vi "Python.vi"() -> ()   [LabVIEW 2014]
uses:
  Controls/Standard Action.ctl
  Controls/StageStates.ctl
  <vilib>/Analysis/baseanly.llb/Mean (DBL).vi
  <vilib>/Analysis/NI_AALBase.lvlib
panel:
  out "queue":string
  out "standard output":string
  out "standard error":string
  in  "port":i32=8900
  in  "hostname":string="localhost"
  out "DM1":dbl[][](graph)
  out "DM0":dbl[][](graph)
  out "Image 2":sgl[][](graph)
  in  "launch_python":bool=TRUE
  in  "script name":string="sensorless.py"
  in  "arguments":string="nelder-mead"
  in  "Run Python":bool
  in  "Exit":bool
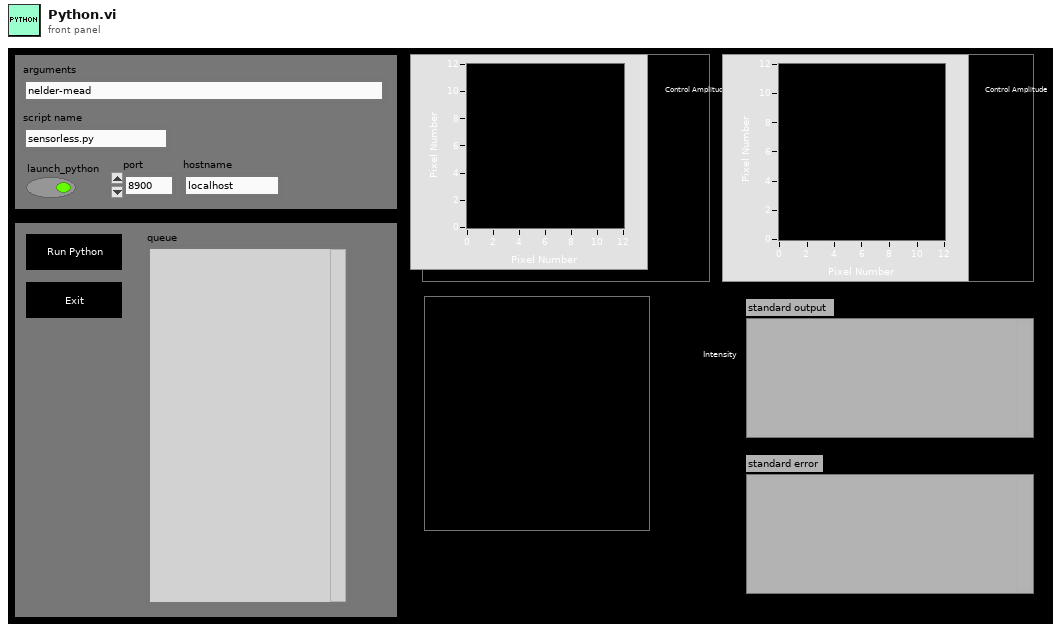
[diagram p1: front panel]
types:
  T1 = typedef "Standard Action.ctl" = enum16{"Read", "Write"}
  T2 = typedef "StageStates.ctl" = enum16{"POSITION", "MVR", "MOVE", "HALT", "ONTARGET", "ERROR", "EXIT", "HOME", "ZEROPOS", "NANOPOS", "QUIT", "ANALOG"}
  T3 = typedef "MirrorModes_DUAL.ctl" = cluster{"Mode":string, "Amplitude":dbl}[][]
  T4 = typedef "Image Acquisition Parameters.ctl" = cluster{"Scan Type":enum16{"Sample Scanning", "Beam Scanning"}, "Scan Mode":enum16{"XY", "XZ", "YZ", "XYZ"}, "Fast Axis Frequency (Hz)":dbl, "Image Format":u16, "Line Accumulations":u16, "Frames Per Capture":u16, "Frames Accumulations":u16, "Image Dimension (um)":dbl[], "Number of Z Steps":u8, "Z Steps Size (um)":dbl, "Pixel Size (nm)":dbl[], "Customized Image Format":dbl[]}
  T5 = typedef "Detectors.ctl" = cluster{"PMT":bool, "Far Red (685/40 nm)":bool, "Orange (624/40 nm)":bool, "Green (525/50 nm)":bool, "Sum All":bool}
  T6 = typedef "Laser Controls.ctl" = cluster{"STED Power (V)":dbl, "STED":bool, "650 nm":bool, "590 nm":bool, "485 nm":bool, "Manual Control":bool}
  T7 = cluster{"dm0":dbl[], "dm1":dbl[], "zcomp":dbl, "stack":sgl[][]}
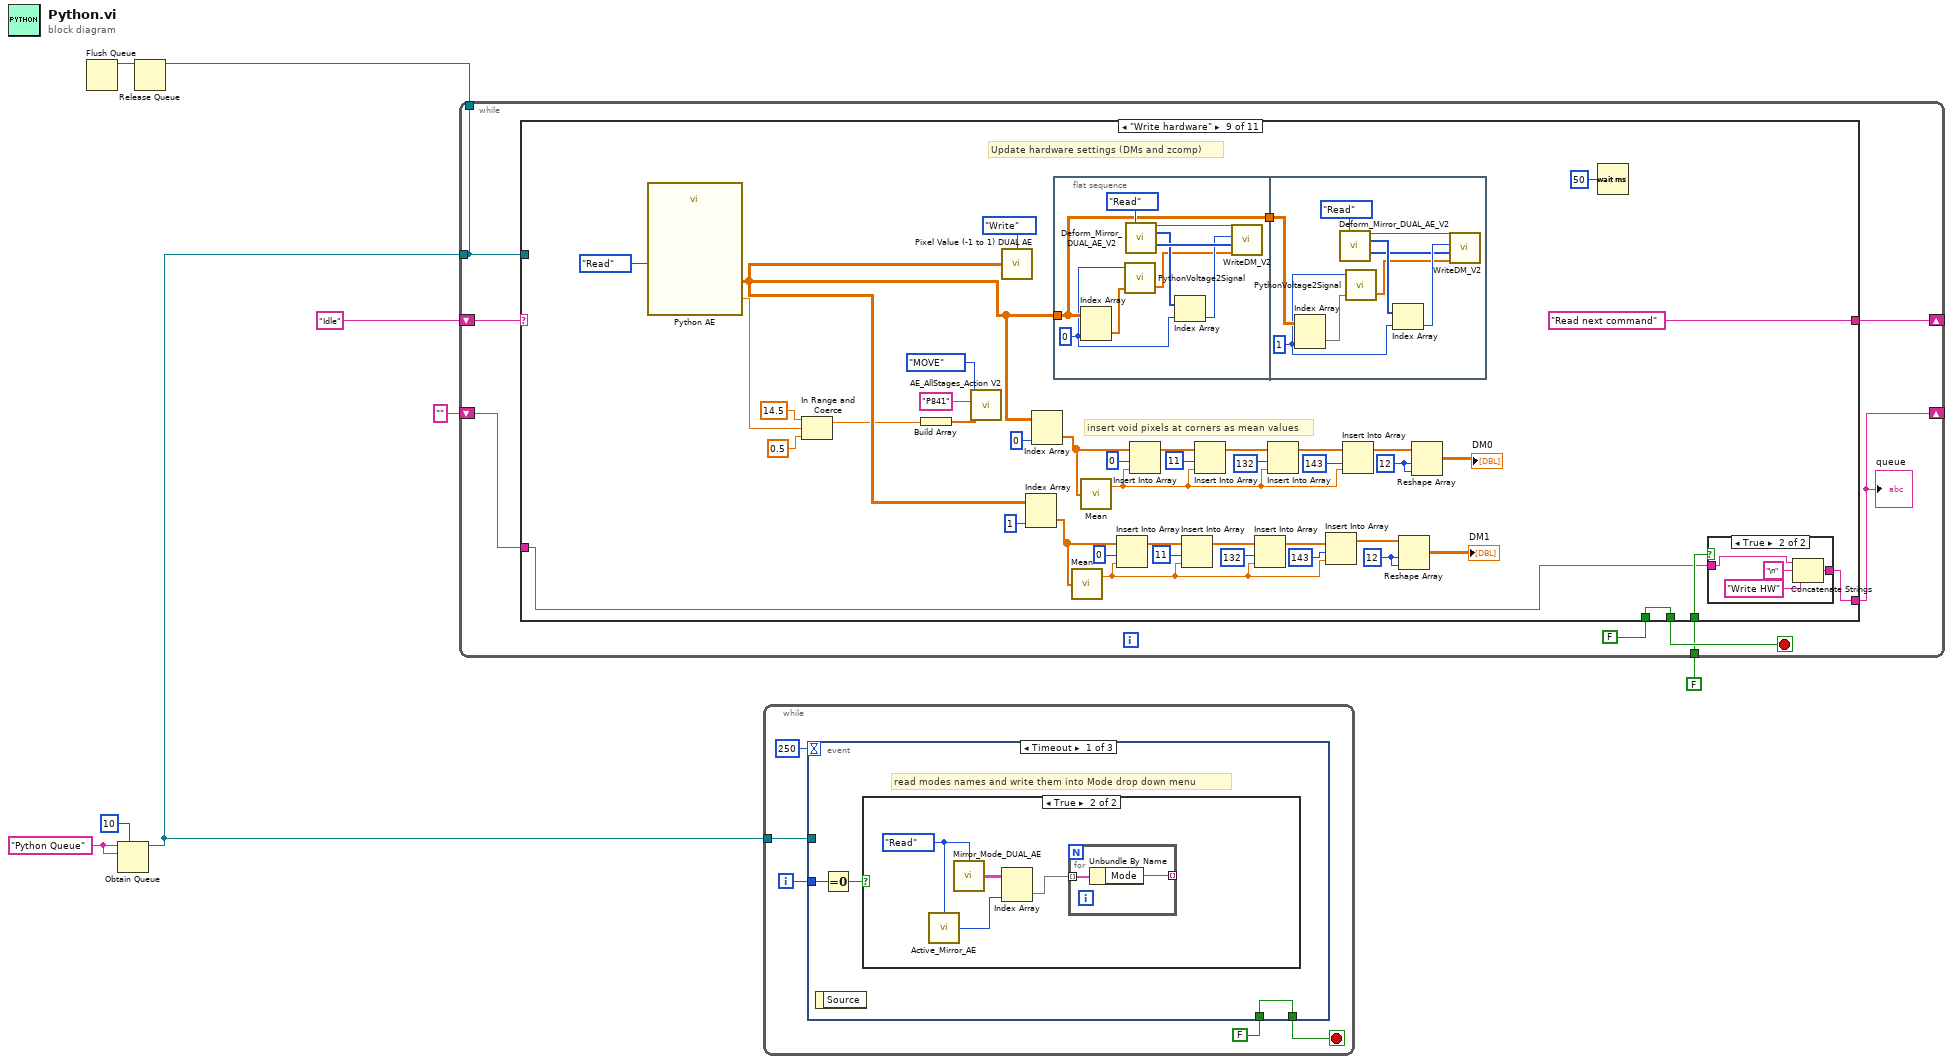
[diagram p0: block diagram]
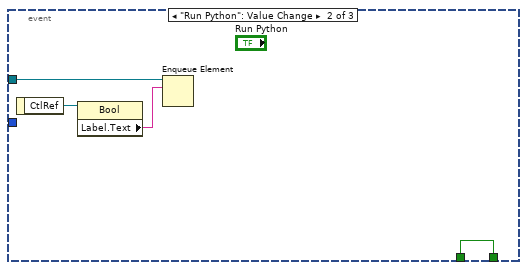
[diagram p3: hidden frame]
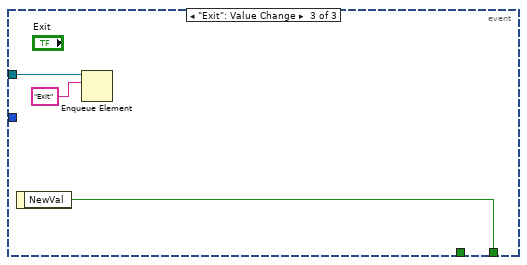
[diagram p4: hidden frame]
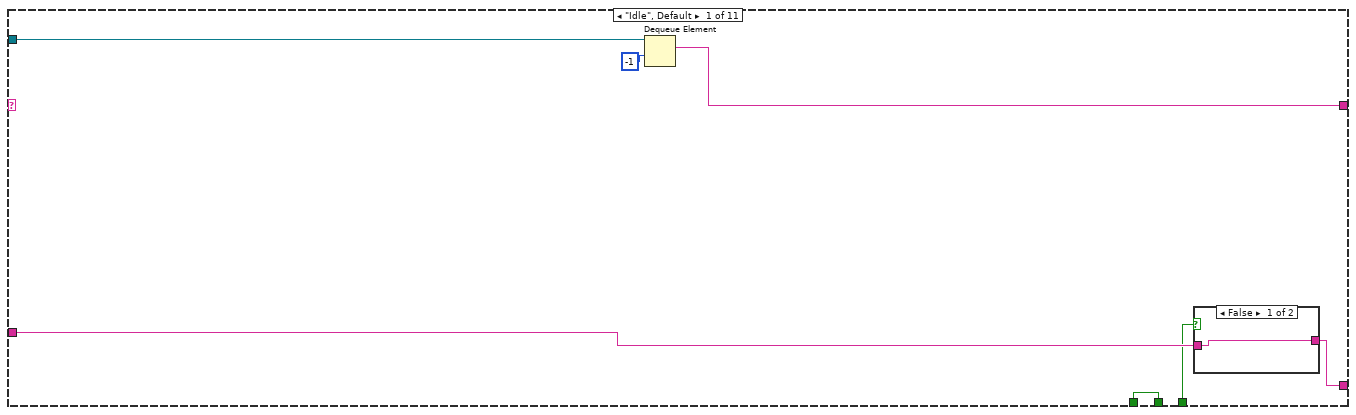
[diagram p5: hidden frame]
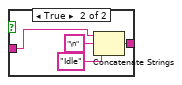
[diagram p6: hidden frame]
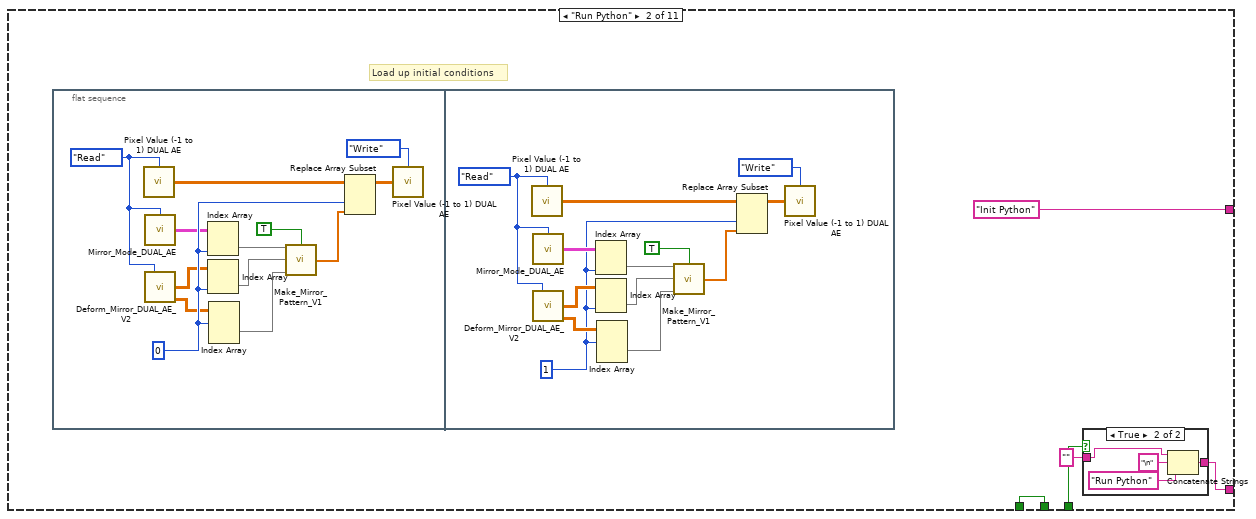
[diagram p7: hidden frame]
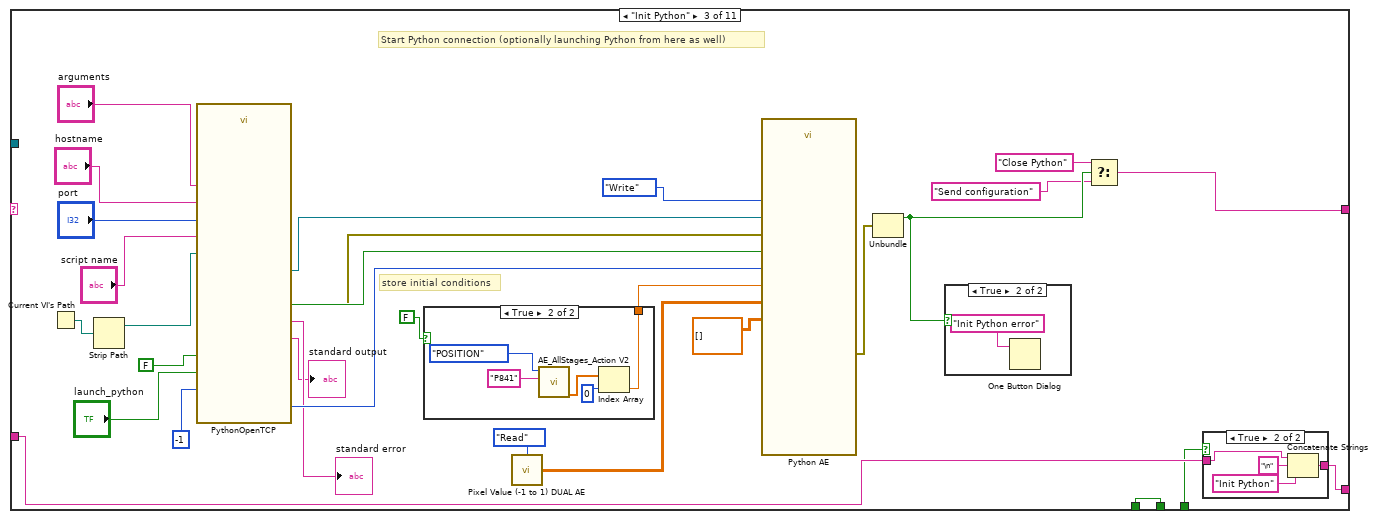
[diagram p9: hidden frame]
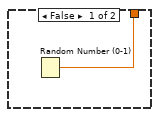
[diagram p11: hidden frame]
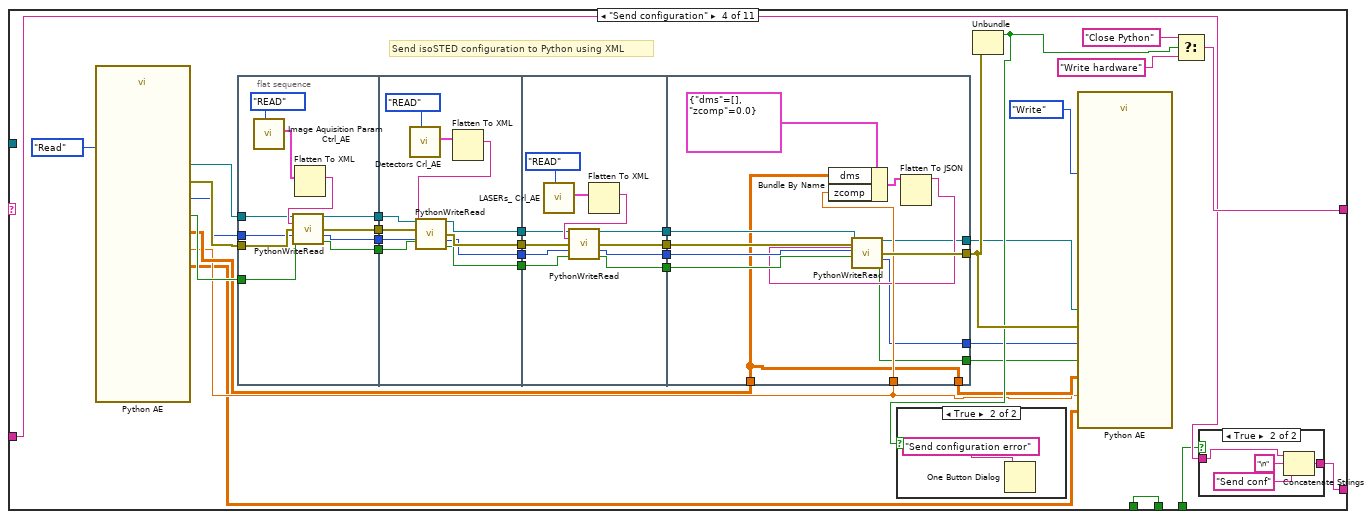
[diagram p13: hidden frame]
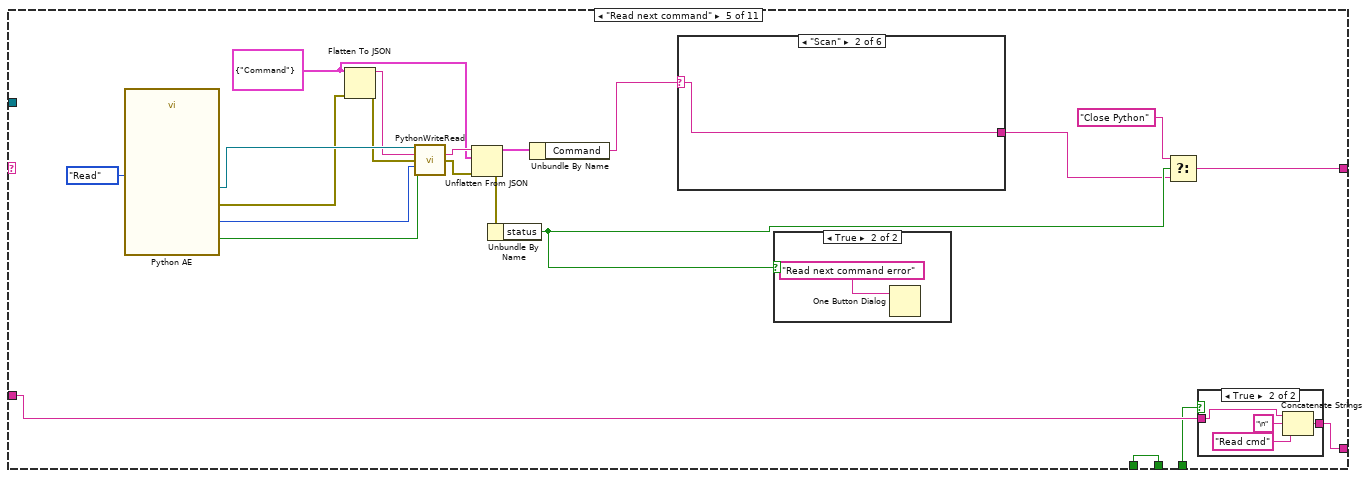
[diagram p16: hidden frame]
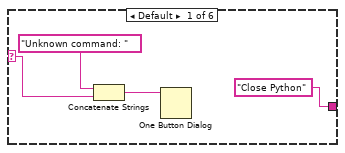
[diagram p18: hidden frame]
diagram:
  w7 = "Python Queue" ("name (unnamed)")
  n1 = Obtain Queue(max queue size (-1, unlimited)=10, name (unnamed)=w7, element data type=w7) -> (queue out=w5:refnum<queue>)  [unwired: 2 in, 2 out]
  n2 = while {
    shift-right: [w11] -> _
    shift-left: "Idle" -> [w13]
    tunnel: w5 -> [w15]
    tunnel: [w15] -> w4
    shift-right: [w10] -> _
    shift-left: "" -> [w12]
    tunnel: FALSE -> [w9]
    stop <- w16 stop-if-true
    n3 = case shown="\"Write hardware\"" w13 {
      tunnel: [w20 w33 w82 w121 w212 w249 w272 w333 w366 w435 TRUE] -> w16
      tunnel: w15 -> [w22 _ _ _ _ _ _ _ _ _ _]
      tunnel: [w21 "Init Python" ("name (unnamed)") w70 w118 w197 w233 "Python pipe" ("name (unnamed)") w334 "Read next command" ("name (unnamed)") "Idle" ("name (unnamed)") "Exit" ("name (unnamed)")] -> w11
      tunnel: FALSE -> [w20 w33 w82 w121 w212 w249 w272 w333 w366 w435 _]
      tunnel: w12 -> [w19 _ w67 w109 w195 w230 w256 w320 w359 w422 w443]
      tunnel: [w17 w31 w66 w108 w194 w231 w258 w321 w358 w421 w444] -> w10
      tunnel: w9 -> [w18 w30 w65 w107 w193 w229 w257 w319 w360 w420 w442]
      frame "Idle", Default {
        n4 = Dequeue Element(queue=w22, timeout in ms (-1)=-1) -> (element=w21:string)  [unwired: 1 in, 3 out]
        n5 = case shown="False" w18 {
          tunnel: [w24 w26] -> w17
          tunnel: w19 -> [w24 w25]
          frame False {
          }
          frame True {
            n6 = Concatenate Strings(w25, "\n" ("string"), "Idle" ("string")) -> (w26:string)
          }
        }
      }
      frame "Run Python" {
        # "Load up initial conditions"
        n7 = flat-sequence {
          frame #0 {
            w51 = 0 ("index (col)")
            w47 = Standard_Action."Read" ("Action")
            n8 = call "Pixel Value (-1 to 1) DUAL AE.vi"("Action"=w47) -> ("Pixel Value (-1 to 1) Out"=w48:dbl[][])  [unwired: 14 in]
            n9 = call "Mirror_Mode_DUAL_AE.vi"("Action"=w47) -> ("Mirror Modes Out"=w44:T3)  [unwired: 14 in]
            n10 = call "Deform_Mirror_DUAL_AE_V2.vi"("Action"=w47) -> ("Flat Files Out"=w42:dbl[][], "Mode Matrix Out"=w40:dbl[][][])  [unwired: 10 in, 3 out]
            n11 = Index Array(array=w44, index (col)=w51) -> (element=w45:cluster{"Mode":string, "Amplitude":dbl}[])  [unwired: 1 in]
            n12 = Index Array(array=w42, index (col)=w51) -> (element=w43:dbl[])  [unwired: 1 in]
            n13 = Index Array(array=w40, index (dim 0)=w51) -> (element=w39:dbl[][])  [unwired: 2 in]
            n14 = call "Make_Mirror_Pattern_V1.vi"("Mirror Modes In"=w45, "Flat On?"=TRUE ("Apply Flat"), "Flat File In"=w43, "Mirror Modes Array"=w39) -> ("Pixel Value U (-1 to 1)"=w49:dbl[])  [unwired: 11 in]
            n15 = Replace Array Subset(array=w48, new element=w49, index (col)=w51) -> (w50:dbl[][])  [unwired: 1 in]
            n16 = call "Pixel Value (-1 to 1) DUAL AE.vi"("Action"=Standard_Action."Write", "Pixel Value (-1 to 1)"=w50) -> ()  [unwired: 13 in, 1 out]
          }
          frame #1 {
            w52 = 1 ("index (col)")
            w56 = Standard_Action."Read" ("Action")
            n17 = call "Pixel Value (-1 to 1) DUAL AE.vi"("Action"=w56) -> ("Pixel Value (-1 to 1) Out"=w55:dbl[][])  [unwired: 14 in]
            n18 = call "Mirror_Mode_DUAL_AE.vi"("Action"=w56) -> ("Mirror Modes Out"=w59:T3)  [unwired: 14 in]
            n19 = call "Deform_Mirror_DUAL_AE_V2.vi"("Action"=w56) -> ("Flat Files Out"=w61:dbl[][], "Mode Matrix Out"=w63:dbl[][][])  [unwired: 10 in, 3 out]
            n20 = Index Array(array=w59, index (col)=w52) -> (element=w58:cluster{"Mode":string, "Amplitude":dbl}[])  [unwired: 1 in]
            n21 = Index Array(array=w61, index (col)=w52) -> (element=w60:dbl[])  [unwired: 1 in]
            n22 = Index Array(array=w63, index (dim 0)=w52) -> (element=w64:dbl[][])  [unwired: 2 in]
            n23 = call "Make_Mirror_Pattern_V1.vi"("Mirror Modes In"=w58, "Flat On?"=TRUE ("Apply Flat"), "Flat File In"=w60, "Mirror Modes Array"=w64) -> ("Pixel Value U (-1 to 1)"=w54:dbl[])  [unwired: 11 in]
            n24 = Replace Array Subset(array=w55, new element=w54, index (col)=w52) -> (w53:dbl[][])  [unwired: 1 in]
            n25 = call "Pixel Value (-1 to 1) DUAL AE.vi"("Action"=Standard_Action."Write", "Pixel Value (-1 to 1)"=w53) -> ()  [unwired: 13 in, 1 out]
          }
        }
        n26 = case shown="True" w30 {
          tunnel: [w34 w36] -> w31
          tunnel: "" -> [w34 w35]
          frame False {
          }
          frame True {
            n27 = Concatenate Strings(w35, "\n" ("string"), "Run Python" ("string")) -> (w36:string)
          }
        }
      }
      frame "Init Python" {
        # "store initial conditions"
        # "Start Python connection (optionally launching Python from here as well)"
        n28 = Current VI's Path() -> (path=w74:path)
        n29 = Strip Path(path=w74) -> (stripped path=w73:path)  [unwired: 1 out]
        n30 = call "PythonOpenTCP.vi"("directory"=w73, "debug"=FALSE, "script name"="script name", "launch_python"="launch_python", "hostname"="hostname", "timeout in"=-1 ("timeout ms (60000)"), "port"="port", "arguments"="arguments") -> ("error out"=w83:errorcluster, "connection out"=w86:refnum<k5>, "standard error"=→"standard error":string, "timeout out"=w84:i32, "run_tcp"=w85:bool, "standard output"=→"standard output":string)  [unwired: 2 in]
        n31 = case shown="True" FALSE {
          tunnel: [w100 w101] -> w77
          frame False {
            n32 = Random Number (0-1)() -> (number: 0 to 1=w100:dbl)
          }
          frame True {
            n33 = call "AE_AllStages_Action V2.vi"("Stage ID"="P841" ("StageID"), "Action"=StageStates."POSITION") -> ("Position Out"=w104:dbl[])  [unwired: 7 in, 2 out]
            n34 = Index Array(array=w104, index=0) -> (element=w101:dbl)
          }
        }
        n35 = call "Pixel Value (-1 to 1) DUAL AE.vi"("Action"=Standard_Action."Read") -> ("Pixel Value (-1 to 1) Out"=w80:dbl[][])  [unwired: 14 in]
        n36 = call "Python AE.vi"("connection"=w86, "error"=w83, "run_tcp"=w85, "timeout"=w84, "u"=w80, "zcomp"=w77, "Action"=Standard_Action."Write", "stack"=sgl[][] []) -> ("error out"=w79:errorcluster)  [unwired: 5 in, 6 out]
        n37 = Unbundle(w79) -> ("status"=w72:bool)  [unwired: 2 out]
        n38 = case shown="True" w72 {
          frame False {
          }
          frame True {
            n39 = One Button Dialog(message="Init Python error") -> ()  [unwired: 1 in, 1 out]
          }
        }
        n40 = Select(t="Close Python", s=w72, f="Send configuration" ("name (unnamed)")) -> (s? t:f=w70:string)
        n41 = case shown="True" w65 {
          tunnel: [w95 w97] -> w66
          tunnel: w67 -> [w95 w96]
          frame False {
          }
          frame True {
            n42 = Concatenate Strings(w96, "\n" ("string"), "Init Python" ("string")) -> (w97:string)
          }
        }
      }
      frame "Send configuration" {
        # "Send isoSTED configuration to Python using XML"
        n43 = call "Python AE.vi"("Action"=Standard_Action."Read") -> ("zcomp out"=w111:dbl, "stack out"=w110:sgl[][], "connection out"=w127:refnum<k5>, "error out"=w126:errorcluster, "u out"=w113:dbl[][], "run_tcp out"=w124:bool, "timeout out"=w125:i32)  [unwired: 12 in]
        n44 = flat-sequence {
          tunnel: [w154] -> w140
          tunnel: [w153] -> w139
          tunnel: [w152] -> w138
          tunnel: [w151] -> w137
          tunnel: w127 -> [w150]
          tunnel: w126 -> [w149]
          tunnel: w125 -> [w148]
          tunnel: w124 -> [w147]
          tunnel: w140 -> [w165]
          tunnel: w139 -> [w164]
          tunnel: w138 -> [w163]
          tunnel: w137 -> [w162]
          tunnel: [w161] -> w136
          tunnel: [w160] -> w135
          tunnel: [w159] -> w134
          tunnel: [w158] -> w133
          tunnel: w136 -> [w176]
          tunnel: w135 -> [w175]
          tunnel: w134 -> [w174]
          tunnel: w133 -> [w173]
          tunnel: [w172] -> w132
          tunnel: [w171] -> w131
          tunnel: [w170] -> w130
          tunnel: [w169] -> w129
          tunnel: w132 -> [w191]
          tunnel: w131 -> [w190]
          tunnel: w130 -> [w189]
          tunnel: w129 -> [w188]
          tunnel: [w187] -> w122
          tunnel: w113 -> [w180]
          tunnel: w111 -> [w186]
          tunnel: [w183] -> w116
          tunnel: [w182] -> w115
          tunnel: [w181] -> w114
          tunnel: [w180] -> w112
          frame #0 {
            n45 = call "Image Aquisition Param Ctrl_AE.vi"("Action"=enum16{"READ", "WRITE"}."READ") -> ("Image Acquisition Parameters Out"=w157:T4)  [unwired: 10 in]
            n46 = Flatten To XML(anything=w157) -> (xml string=w155:string)
            n47 = call "PythonWriteRead.vi"("connection in"=w150, "string in"=w155, "error in"=w149, "timeout in"=w148, "run_tcp in"=w147) -> ("connection out"=w154:refnum<k5>, "error out"=w153:errorcluster, "timeout out"=w152:i32, "run_tcp out"=w151:bool)  [unwired: 6 in, 1 out]
          }
          frame #1 {
            n48 = call "Detectors Crl_AE.vi"("Action"=enum16{"READ", "WRITE"}."READ") -> ("Detectors Parameters Out"=w167:T5)  [unwired: 10 in]
            n49 = Flatten To XML(anything=w167) -> (xml string=w166:string)
            n50 = call "PythonWriteRead.vi"("connection in"=w165, "string in"=w166, "error in"=w164, "timeout in"=w163, "run_tcp in"=w162) -> ("connection out"=w161:refnum<k5>, "error out"=w160:errorcluster, "timeout out"=w159:i32, "run_tcp out"=w158:bool)  [unwired: 6 in, 1 out]
          }
          frame #2 {
            n51 = call "LASERs_ Crl_AE.vi"("Action"=enum16{"READ", "WRITE"}."READ") -> ("Detectors Parameters Out"=w179:T6)  [unwired: 10 in]
            n52 = Flatten To XML(anything=w179) -> (xml string=w177:string)
            n53 = call "PythonWriteRead.vi"("connection in"=w176, "string in"=w177, "error in"=w175, "timeout in"=w174, "run_tcp in"=w173) -> ("connection out"=w172:refnum<k5>, "error out"=w171:errorcluster, "timeout out"=w170:i32, "run_tcp out"=w169:bool)  [unwired: 6 in, 1 out]
          }
          frame #3 {
            n54 = Bundle By Name(cluster=cluster{"dms":dbl[][], "zcomp":dbl} {"dms"=[], "zcomp"=0.0} ("input cluster"), "dms"=w180, "zcomp"=w186) -> (w185:cluster{"dms":dbl[][], "zcomp":dbl})
            n55 = Flatten To JSON(anything=w185) -> (JSON string=w184:string)  [unwired: 2 in, 1 out]
            n56 = call "PythonWriteRead.vi"("connection in"=w191, "string in"=w184, "error in"=w190, "timeout in"=w189, "run_tcp in"=w188) -> ("connection out"=w183:refnum<k5>, "error out"=w187:errorcluster, "timeout out"=w182:i32, "run_tcp out"=w181:bool)  [unwired: 6 in, 1 out]
          }
        }
        n57 = Unbundle(w122) -> ("status"=w117:bool)  [unwired: 2 out]
        n58 = case shown="True" w117 {
          frame False {
          }
          frame True {
            n59 = One Button Dialog(message="Send configuration error") -> ()  [unwired: 1 in, 1 out]
          }
        }
        n60 = call "Python AE.vi"("connection"=w116, "error"=w122, "run_tcp"=w114, "timeout"=w115, "u"=w112, "zcomp"=w111, "Action"=Standard_Action."Write", "stack"=w110) -> ()  [unwired: 5 in, 7 out]
        n61 = Select(t="Close Python", s=w117, f="Write hardware" ("name (unnamed)")) -> (s? t:f=w118:string)
        n62 = case shown="True" w107 {
          tunnel: [w141 w143] -> w108
          tunnel: w109 -> [w141 w142]
          frame False {
          }
          frame True {
            n63 = Concatenate Strings(w142, "\n" ("string"), "Send conf" ("string")) -> (w143:string)
          }
        }
      }
      frame "Read next command" {
        w204 = cluster{"Command":string} {"Command"="Command"} ("input cluster")
        n64 = call "Python AE.vi"("Action"=Standard_Action."Read") -> ("connection out"=w211:refnum<k5>, "error out"=w209:errorcluster, "run_tcp out"=w206:bool, "timeout out"=w207:i32)  [unwired: 12 in, 3 out]
        n65 = Flatten To JSON(anything=w204, error in (no error)=w209) -> (JSON string=w210:string, 11:w208:errorcluster)  [unwired: 1 in]
        n66 = call "PythonWriteRead.vi"("connection in"=w211, "string in"=w210, "error in"=w208, "timeout in"=w207, "run_tcp in"=w206) -> ("string out"=w205:string, "error out"=w203:errorcluster)  [unwired: 6 in, 3 out]
        n67 = Unflatten From JSON(JSON string=w205, type and defaults=w204, error in (no error)=w203) -> (value=w196:cluster{"Command":string}, error out=w202:errorcluster)  [unwired: 4 in]
        n68 = Unbundle By Name(w202) -> ("status"=w200:bool)
        n69 = Unbundle By Name(w196) -> ("Command"=w201:string)
        n70 = case shown="\"Scan\"" w201 {
          selector: w201 -> [w219 w223 w224 w225 w226 _]
          tunnel: ["Close Python" ("t") w223 w224 w225 w226 "Close Python" ("t")] -> w198
          frame Default {
            n71 = Concatenate Strings("Unknown command: " ("message"), w219) -> (w221:string)
            n72 = One Button Dialog(message=w221) -> ()  [unwired: 1 in, 1 out]
          }
          frame "Scan" {
          }
          frame "Image acquisition params" {
          }
          frame "Detectors params" {
          }
          frame "Laser params" {
          }
          frame "Stop" {
          }
        }
        n73 = case shown="True" w200 {
          frame False {
          }
          frame True {
            n74 = One Button Dialog(message="Read next command error") -> ()  [unwired: 1 in, 1 out]
          }
        }
        n75 = Select(t="Close Python" ("f"), s=w200, f=w198) -> (s? t:f=w197:string)
        n76 = case shown="True" w193 {
          tunnel: [w214 w216] -> w194
          tunnel: w195 -> [w214 w215]
          frame False {
          }
          frame True {
            n77 = Concatenate Strings(w215, "\n" ("string"), "Read cmd" ("string")) -> (w216:string)
          }
        }
      }
      frame "Image acquisition params" {
        # "Send isoSTED configuration to Python using XML"
        n78 = call "Python AE.vi"("Action"=Standard_Action."Read") -> ("connection out"=w247:refnum<k5>, "error out"=w246:errorcluster, "run_tcp out"=w244:bool, "timeout out"=w245:i32)  [unwired: 12 in, 3 out]
        n79 = call "Image Aquisition Param Ctrl_AE.vi"("Action"=enum16{"READ", "WRITE"}."READ") -> ("Image Acquisition Parameters Out"=w241:T4)  [unwired: 10 in]
        n80 = Flatten To XML(anything=w241) -> (xml string=w238:string)
        n81 = call "PythonWriteRead.vi"("connection in"=w247, "string in"=w238, "error in"=w246, "timeout in"=w245, "run_tcp in"=w244) -> ("string out"=w243:string, "error out"=w242:errorcluster)  [unwired: 6 in, 3 out]
        n82 = Unflatten From XML(xml string=w243, type=w241, error in (no error)=w242) -> (value=w236:T4, error out=w240:errorcluster)
        n83 = call "Image Aquisition Param Ctrl_AE.vi"("Action"=enum16{"READ", "WRITE"}."WRITE", "Image Acquisition Parameters In"=w236) -> ()  [unwired: 9 in, 1 out]
        n84 = Unbundle(w240) -> ("status"=w232:bool)  [unwired: 2 out]
        n85 = case shown="True" w232 {
          frame False {
          }
          frame True {
            n86 = One Button Dialog(message="Image acquisition params error") -> ()  [unwired: 1 in, 1 out]
          }
        }
        n87 = Select(t="Close Python", s=w232, f="Read next command" ("name (unnamed)")) -> (s? t:f=w233:string)
        n88 = case shown="True" w229 {
          tunnel: [w250 w252] -> w231
          tunnel: w230 -> [w250 w251]
          frame False {
          }
          frame True {
            n89 = Concatenate Strings(w251, "\n" ("string"), "Acq params" ("string")) -> (w252:string)
          }
        }
      }
      frame "Scan" {
        w277 = "Acquisition" ("name (unnamed)")
        # "Perform scan"
        n90 = Obtain Queue(max queue size (-1, unlimited)=10, name (unnamed)=w277, element data type=w277) -> (queue out=w274:refnum<queue>, created new?=w280:bool)  [unwired: 2 in, 1 out]
        n91 = Obtain Notifier(name (unnamed)="Running", notification data type=TRUE) -> (notifier out=w275:refnum<notifier>, created new?=w281:bool)  [unwired: 2 in, 1 out]
        n92 = Or(x=w280, y=w281) -> (x .or. y?=w282:bool)
        n93 = call "AE_AllStages_Action V2.vi"("Stage ID"="P841" ("StageID"), "Action"=StageStates."POSITION") -> ("Position Out"=w269:dbl[])  [unwired: 7 in, 2 out]
        n94 = case shown="False" w282 {
          tunnel: w274 -> [w291 _]
          tunnel: w275 -> [w289 _]
          tunnel: [w288 sgl[][] [] ("Value")] -> w260
          frame False {
            n95 = call "Graph Ref AE.vi"("Action"=enum16{"READ", "WRITE"}."READ") -> ("Graph Ref Out"=w299:refnum<vi>[])  [unwired: 10 in]
            n96 = Send Notification(notification=FALSE, notifier=w289) -> (notifier out=w294:refnum<notifier>, error out=w293:errorcluster)  [unwired: 1 in]
            n97 = Enqueue Element(queue=w291, element="Capture", error in (no error)=w293) -> (queue out=w295:refnum<queue>)  [unwired: 1 in, 2 out]
            n98 = Index Array(array=w299, index=0) -> (element=w301:refnum<vi>)
            n99 = while {
              tunnel: w294 -> [w307]
              tunnel: [w305] -> w296
              tunnel: w295 -> [w305]
              tunnel: [w304] -> w302
              tunnel: w301 -> [w304]
              stop <- w306 stop-if-true
              n100 = Get Notifier Status(notifier=w307) -> (current notification=w306:bool)  [unwired: 1 in, 4 out]
              n101 = Wait (ms)(milliseconds to wait=u32 0) -> ()  [unwired: 1 out]
            }
            n102 = property class="IntGraph (strict)"(reference=w302) -> ("Value"=w288:sgl[][])  [unwired: 1 in, 2 out]
            "Image 2" <- w288
            n103 = Enqueue Element(queue=w296, element="Stop Acquisition" ("f")) -> ()  [unwired: 2 in, 3 out]
          }
          frame True {
            # "Acquisition and Running were not found"
            n104 = One Button Dialog(message="Acquisition queue Not Found") -> ()  [unwired: 1 in, 1 out]
          }
        }
        n105 = Index Array(array=w269, index=0) -> (element=w259:dbl)
        n106 = call "Python AE.vi"("Action"=Standard_Action."Read") -> ("connection out"=w265:refnum<k5>, "error out"=w264:errorcluster, "u out"=w261:dbl[][], "run_tcp out"=w262:bool, "timeout out"=w263:i32)  [unwired: 12 in, 2 out]
        n107 = call "Python AE.vi"("connection"=w265, "error"=w264, "run_tcp"=w262, "timeout"=w263, "u"=w261, "zcomp"=w259, "Action"=Standard_Action."Write", "stack"=w260) -> ()  [unwired: 5 in, 7 out]
        n108 = case shown="True" w257 {
          tunnel: [w283 w285] -> w258
          tunnel: w256 -> [w283 w284]
          frame False {
          }
          frame True {
            n109 = Concatenate Strings(w284, "\n" ("string"), "Scan" ("string")) -> (w285:string)
          }
        }
      }
      frame "Python pipe" {
        w346 = T7 {"dm0"=[], "dm1"=[], "zcomp"=0.0, "stack"=[]} ("input cluster")
        # "Pipe scan data to Python using JSON"
        n110 = call "Python AE.vi"("Action"=Standard_Action."Read") -> ("zcomp out"=w325:dbl, "stack out"=w324:sgl[][], "connection out"=w318:refnum<k5>, "error out"=w322:errorcluster, "u out"=w328:dbl[][], "run_tcp out"=w314:bool, "timeout out"=w316:i32)  [unwired: 12 in]
        n111 = Index Array(array=w328, index (col)=1 ("disabled index (col)")) -> (element=w326:dbl[])  [unwired: 1 in]
        n112 = Index Array(array=w328, index (col)=0 ("disabled index (col)")) -> (element=w327:dbl[])  [unwired: 1 in]
        n113 = Bundle By Name(cluster=w346, "dm0"=w327, "dm1"=w326, "zcomp"=w325, "stack"=w324) -> (w345:T7)
        n114 = Flatten To JSON(anything=w345, error in (no error)=w322) -> (JSON string=w341:string, 11:w340:errorcluster)  [unwired: 1 in]
        n115 = call "PythonWriteRead.vi"("connection in"=w318, "string in"=w341, "error in"=w340, "timeout in"=w316, "run_tcp in"=w314) -> ("connection out"=w317:refnum<k5>, "string out"=w339:string, "error out"=w347:errorcluster, "timeout out"=w315:i32, "run_tcp out"=w313:bool)  [unwired: 6 in]
        n116 = Unflatten From JSON(JSON string=w339, type and defaults=w346, error in (no error)=w347) -> (value=w344:T7, error out=w330:errorcluster)  [unwired: 4 in]
        n117 = Unbundle By Name(w344) -> ("dm0"=w338:dbl[], "dm1"=w337:dbl[], "zcomp"=w331:dbl, "stack"=w323:sgl[][])
        n118 = Unbundle By Name(w330) -> ("status"=w312:bool)
        n119 = Build Array(w338, w337) -> (w311:dbl[][])
        n120 = Transpose 2D Array(2D array=w311) -> (transposed array=w310:dbl[][])
        n121 = case shown="True" w312 {
          frame False {
          }
          frame True {
            n122 = One Button Dialog(message="Python pipe error") -> ()  [unwired: 1 in, 1 out]
          }
        }
        n123 = call "Python AE.vi"("connection"=w317, "error"=w330, "run_tcp"=w313, "timeout"=w315, "u"=w310, "zcomp"=w331, "Action"=Standard_Action."Write", "stack"=w323) -> ()  [unwired: 5 in, 7 out]
        n124 = Select(t="Close Python", s=w312, f="Write hardware") -> (s? t:f=w334:string)
        n125 = case shown="True" w319 {
          tunnel: [w348 w350] -> w321
          tunnel: w320 -> [w348 w349]
          frame False {
          }
          frame True {
            n126 = Concatenate Strings(w349, "\n" ("string"), "Pipe" ("string")) -> (w350:string)
          }
        }
      }
      frame "Write hardware" {
        w370 = 12 ("dimension size")
        w380 = 12 ("dimension size")
        # "Update hardware settings (DMs and zcomp)"
        # "insert void pixels at corners as mean values"
        n127 = call "Python AE.vi"("Action"=Standard_Action."Read") -> ("zcomp out"=w364:dbl, "u out"=w367:dbl[][])  [unwired: 12 in, 5 out]
        n128 = In Range and Coerce(upper limit=14.5, x=w364, lower limit=0.5) -> (coerced(x)=w363:dbl)  [unwired: 1 out]
        n129 = Build Array(w363) -> (w393:dbl[])
        n130 = call "AE_AllStages_Action V2.vi"("Positions"=w393, "Stage ID"="P841" ("StageID"), "Action"=StageStates."MOVE") -> ()  [unwired: 6 in, 3 out]
        n131 = call "Pixel Value (-1 to 1) DUAL AE.vi"("Action"=Standard_Action."Write", "Pixel Value (-1 to 1)"=w367) -> ()  [unwired: 13 in, 1 out]
        n132 = Index Array(array=w367, index (col)=1 ("disabled index (col)")) -> (element=w356:dbl[])  [unwired: 1 in]
        n133 = Index Array(array=w367, index (col)=0 ("disabled index (col)")) -> (element=w357:dbl[])  [unwired: 1 in]
        n134 = flat-sequence {
          tunnel: w367 -> [w405]
          tunnel: [w405] -> w391
          tunnel: w391 -> [w414]
          frame #0 {
            w404 = 0 ("disabled index (col)")
            n135 = Index Array(array=w405, index (col)=w404) -> (element=w403:dbl[])  [unwired: 1 in]
            n136 = call "PythonVoltage2Signal.vi"("Control Signal In (-1~1)"=w403, "DM #"=w404) -> ("Voltage Out (0~Max. Vol.)"=w402:dbl[])  [unwired: 1 in, 1 out]
            n137 = call "Deform_Mirror_DUAL_AE_V2.vi"("Action"=Standard_Action."Read") -> ("Refnum Out"=w410:refnum<k7>, "IDs Out"=w407:i32[], "Multi Map Data Out"=w409:i32[])  [unwired: 10 in, 2 out]
            n138 = Index Array(array=w407, index=w404) -> (element=w406:i32)
            n139 = call "WriteDM_V2.vi"("reference in"=w410, "nDevId"=w406, "MultiDM  Mapping"=w409, "Voltage Array in"=w402) -> ()  [unwired: 2 in, 2 out]
          }
          frame #1 {
            w413 = 1 ("disabled index (col)")
            n140 = Index Array(array=w414, index (col)=w413) -> (element=w412:dbl[])  [unwired: 1 in]
            n141 = call "Deform_Mirror_DUAL_AE_V2.vi"("Action"=Standard_Action."Read") -> ("Refnum Out"=w415:refnum<k7>, "IDs Out"=w418:i32[], "Multi Map Data Out"=w416:i32[])  [unwired: 10 in, 2 out]
            n142 = call "PythonVoltage2Signal.vi"("Control Signal In (-1~1)"=w412, "DM #"=w413) -> ("Voltage Out (0~Max. Vol.)"=w411:dbl[])  [unwired: 1 in, 1 out]
            n143 = Index Array(array=w418, index=w413) -> (element=w419:i32)
            n144 = call "WriteDM_V2.vi"("reference in"=w415, "nDevId"=w419, "MultiDM  Mapping"=w416, "Voltage Array in"=w411) -> ()  [unwired: 2 in, 2 out]
          }
        }
        n145 = call-poly <vilib>:"Mean.vi"("X"=w356) -> ("mean"=w354:dbl)  [unwired: 1 out]
        n146 = call-poly <vilib>:"Mean.vi"("X"=w357) -> ("mean"=w355:dbl)  [unwired: 1 out]
        n147 = Insert Into Array(array=w356, index=0, new element=w354) -> (w376:dbl[])
        n148 = Insert Into Array(array=w357, index=0, new element=w355) -> (w386:dbl[])
        n149 = Insert Into Array(array=w376, index=11, new element=w354) -> (w374:dbl[])
        n150 = Insert Into Array(array=w386, index=11, new element=w355) -> (w384:dbl[])
        n151 = Insert Into Array(array=w374, index=132, new element=w354) -> (w372:dbl[])
        n152 = Insert Into Array(array=w384, index=132, new element=w355) -> (w382:dbl[])
        n153 = Insert Into Array(array=w372, index=143, new element=w354) -> (w379:dbl[])
        n154 = Insert Into Array(array=w382, index=143, new element=w355) -> (w389:dbl[])
        n155 = Reshape Array(w379, w370, w370) -> (→"DM1":dbl[][])
        n156 = Reshape Array(w389, w380, w380) -> (→"DM0":dbl[][])
        n157 = Wait (ms)(milliseconds to wait=u32 50) -> ()  [unwired: 1 out]
        n158 = case shown="True" w360 {
          tunnel: [w397 w399] -> w358
          tunnel: w359 -> [w397 w398]
          frame False {
          }
          frame True {
            n159 = Concatenate Strings(w398, "\n" ("string"), "Write HW" ("string")) -> (w399:string)
          }
        }
      }
      frame "Close Python" {
        n160 = call "Python AE.vi"("Action"=Standard_Action."Read") -> ("connection out"=w433:refnum<k5>, "error out"=w431:errorcluster, "run_tcp out"=w432:bool)  [unwired: 12 in, 4 out]
        n161 = call "PythonCloseTCP.vi"("connection in"=w433, "run_tcp"=w432, "error in"=w431) -> ()  [unwired: 12 in, 1 out]
        n162 = call "Python AE.vi"("connection"=refnum<k5> refnum, "error"=errorcluster {"status"=FALSE, "code"=0, "source"=""}, "run_tcp"=FALSE, "timeout"=-1, "u"=dbl[][] [], "zcomp"=0.0, "Action"=Standard_Action."Write", "stack"=sgl[][] []) -> ()  [unwired: 5 in, 7 out]
        n163 = case shown="True" w420 {
          tunnel: [w437 w439] -> w421
          tunnel: w422 -> [w437 w438]
          frame False {
          }
          frame True {
            n164 = Concatenate Strings(w438, "\n" ("string"), "Close Python" ("string")) -> (w439:string)
          }
        }
      }
      frame "Exit" {
        n165 = case shown="True" w442 {
          tunnel: [w447 w449] -> w444
          tunnel: w443 -> [w447 w448]
          frame False {
          }
          frame True {
            n166 = Concatenate Strings(w448, "\n" ("string"), "Exit" ("string")) -> (w449:string)
          }
        }
      }
    }
    "queue" <- w10
  }
  n167 = Flush Queue(queue=w4) -> (queue out=w3:refnum<queue>)  [unwired: 1 in, 2 out]
  n168 = Release Queue(queue=w3) -> ()  [unwired: 2 in, 3 out]
  n169 = while {
    tunnel: w5 -> [w456]
    i -> [w453]
    stop <- w455 stop-if-true
    n170 = event shown="[0] Timeout" {
      selector: _ -> [_ _ _]
      dyn-events: _ -> [_ _ _]
      timeout: 250 -> [_ _ _]
      tunnel: w456 -> [_ w468 w472]
      tunnel: [w459 w466 w470] -> w455
      tunnel: FALSE -> [w459 w466 _]
      tunnel: w453 -> [w458 _ _]
      event Timeout {
        # "read modes names and write them into Mode drop down menu"
        n171 = event-data() -> ()  [unwired: 1 in, 1 out]
        n172 = Equal To 0?(x=w458) -> (x = 0?=w457:bool)
        n173 = case shown="True" w457 {
          frame False {
          }
          frame True {
            w463 = Standard_Action."Read" ("Action")
            n174 = call "Active_Mirror_AE.vi"("Action"=w463) -> ("Active Mirror"=w460:i32)  [unwired: 14 in]
            n175 = call "Mirror_Mode_DUAL_AE.vi"("Action"=w463) -> ("Mirror Modes Out"=w462:T3)  [unwired: 14 in]
            n176 = Index Array(array=w462, index (col)=w460) -> (element=w461:cluster{"Mode":string, "Amplitude":dbl}[])  [unwired: 1 in]
            n177 = for {
              tunnel: w461 -> [w465] mode=indexing
              tunnel: [w464] -> _ mode=indexing
              n178 = Unbundle By Name(w465) -> ("Mode"=w464:string)
            }
          }
        }
      }
      event "Run Python": Value Change {
        n179 = event-data() -> ("CtlRef"=w467:refnum<vi>)  [unwired: 1 in]
        n180 = property class="Bool"(reference=w467) -> ("Label.Text"=w469:string)  [unwired: 1 in, 2 out]
        n181 = Enqueue Element(queue=w468, element=w469) -> ()  [unwired: 2 in, 3 out]
      }
      event "Exit": Value Change {
        n182 = event-data() -> ("NewVal"=w470:bool)  [unwired: 1 in]
        n183 = Enqueue Element(queue=w472, element="Exit") -> ()  [unwired: 2 in, 3 out]
      }
    }
  }
